vi "MG3700 Frequency_user.vi"(5 "Units (Hz)":T1, 6 "Error in (no error)":errorcluster, 7 "Frequency (250000)":dbl=250000.0 format="%#.5f", 8 "Set/Get (Set)":T2, 9 "VISA In":refnum<visa-resource-name>) -> (0 "Error out":errorcluster, 1 "Error code":i32, 2 "Frequency out":dbl format="%#.9f", 3 "VISA Out":refnum<visa-resource-name>, 4 "Units out":T1)   [LabVIEW 2015]
doc: "Function: Sets a frequency."
uses:
  Controls/Set_Get.ctl
  Controls/Hz_KHz_MHz_GHz.ctl
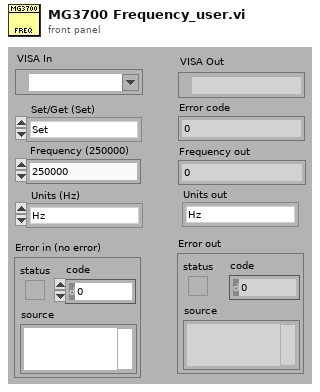
[diagram p1: front panel]
types:
  T1 = typedef "Hz_KHz_MHz_GHz.ctl" = enum16{"Hz", "KHz", "MHz", "GHz"}
  T2 = typedef "Set_Get.ctl" = enum16{"Set", "Get"}
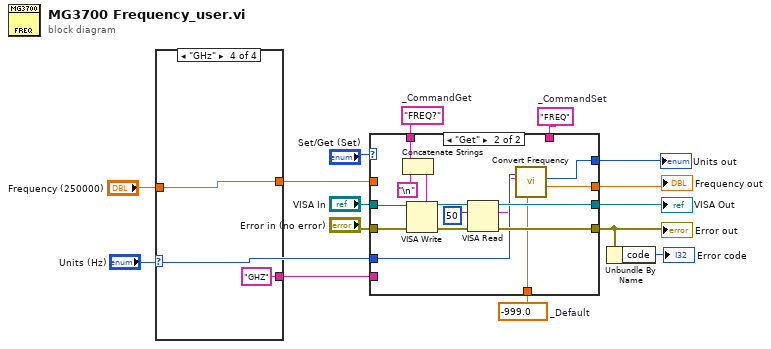
[diagram p0: block diagram]
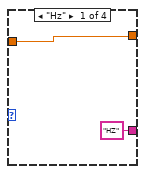
[diagram p2: hidden frame]
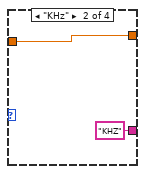
[diagram p3: hidden frame]
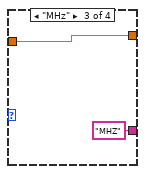
[diagram p4: hidden frame]
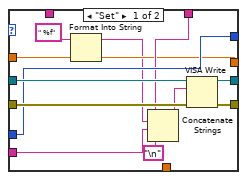
[diagram p5: hidden frame]
diagram:
  w6 = "FREQ"  # _CommandSet
  w8 = -999.0  # _Default
  w7 = "FREQ?"  # _CommandGet
  n1 = case shown="\"GHz\"" "Units (Hz)" {
    tunnel: "Frequency (250000)" -> [w16 w18 w20 w22]
    tunnel: [w16 w18 w20 w22] -> w3
    tunnel: ["HZ" "KHZ" "MHZ" "GHZ"] -> w1
    frame "Hz" {
    }
    frame "KHz" {
    }
    frame "MHz" {
    }
    frame "GHz" {
    }
  }
  n2 = case shown="\"Get\"" "Set/Get (Set)" {
    tunnel: "VISA In" -> [w35 w50]
    tunnel: [w34 w44] -> w14
    tunnel: [w33 w45] -> w12
    tunnel: "Error in (no error)" -> [w32 w49]
    tunnel: [w25 w38] -> w9
    tunnel: "Units (Hz)" -> [w29 w39]
    tunnel: w8 -> [_ w40]
    tunnel: w7 -> [_ w41]
    tunnel: w6 -> [w27 _]
    tunnel: [w29 w37] -> w5
    tunnel: w3 -> [w25 _]
    tunnel: w1 -> [w28 _]
    frame "Set" {
      n3 = Format Into String(format string=" %f" ("Format String"), w25) -> (resulting string=w24:string)  [unwired: 2 in, 1 out]
      n4 = Concatenate Strings(w27, w24, w28, "\n") -> (w31:string)
      n5 = VISA Write(VISA resource name=w35, write buffer=w31, error in (no error)=w32) -> (VISA resource name out=w33:refnum<visa-resource-name>, error out=w34:errorcluster)  [unwired: 1 out]
    }
    frame "Get" {
      n6 = Concatenate Strings(w41, "\n") -> (w42:string)
      n7 = VISA Write(VISA resource name=w50, write buffer=w42, error in (no error)=w49) -> (VISA resource name out=w48:refnum<visa-resource-name>, error out=w47:errorcluster)  [unwired: 1 out]
      n8 = VISA Read(VISA resource name=w48, byte count=u32 50 ("byte count (0)"), error in (no error)=w47) -> (VISA resource name out=w45:refnum<visa-resource-name>, read buffer=w36:string, error out=w44:errorcluster)  [unwired: 1 out]
      n9 = call "Convert Frequency.vi"("Default (-999.00)"=w40, "Units (Hz)"=w39, "String"=w36) -> ("Frequency"=w38:dbl, "Units out"=w37:T1)  [unwired: 7 in]
    }
  }
  "VISA Out" <- w12
  "Error out" <- w14
  "Frequency out" <- w9
  "Units out" <- w5
  n10 = Unbundle By Name(w14) -> ("code"=→"Error code":i32)
